vi "Global_Configurations.vi"() -> ()   [LabVIEW 2019]
panel:
  in  "LabVIEW Port":u16=3363 caption="SSE_frequency"
  in  "LabVIEW Host":string="localhost"
  in  "Session_timeout":u32=14400000
  in  "Reconnect_session_timeout":u32=12000
  in  "SSE_frequency":u32=200
  in  "Timeout_to abort_a_nonresponding_VI":u32=5000
  in  "License":cluster{"ID":string, "Number":string}
  in  "Access-Control-Allow-Credentials":string(combo)="true"
  out "VI_Disconnections":u8[](array[numeric])
  out "VI_Connections":u8[](array[numeric])
  in  "Access-Control-Allow-Origin":string
  in  "Default Experience":string="TestOK"
  in  "Base URL":string
  in  "Experiments":T1(array[cluster])=[{"Path"=path "../Private/TestOK.vi", "Name"="TestOK", "Authors"="D.Chaos", "Keywords"="Test", "Description"="TestOK.vi is used to test the correct execution of a well-defined vi through RIP", "Cameras"=[{"Base URL"="http://camera1_ip", "Path"="/axis-cgi/mjpg/video.cgi", "Name"="Camera 1"}, {"Base URL"="http://camera2_ip", "Path"="/axis-cgi/mjpg/video.cgi", "Name"="Camera 2"}], "Sampling"=[{"Sampled Variable"="t", "Delta"=5.0}], "Sampling Freq"=200}, {"Path"=path "C:/Users/Luis de la Torre/Documents/TestOK.vi", "Name"="TestOK2", "Authors"="D.Chaos", "Keywords"="Test", "Description"="TestOK.vi is used to test the correct execution of a well-defined vi through RIP", "Cameras"=[{"Base URL"="http://camera1_ip", "Path"="/axis-cgi/mjpg/video.cgi", "Name"="Camera 1"}, {"Base URL"="http://camera2_ip", "Path"="/axis-cgi/mjpg/video.cgi", "Name"="Camera 2"}], "Sampling"=[{"Sampled Variable"="t", "Delta"=5.0}], "Sampling Freq"=200}, {"Path"=path "C:/TestOK.vi", "Name"="TestOK3", "Authors"="D.Chaos", "Keywords"="Test", "Description"="TestOK.vi is used to test the correct execution of a well-defined vi through RIP", "Cameras"=[{"Base URL"="http://camera1_ip", "Path"="/axis-cgi/mjpg/video.cgi", "Name"="Camera 1"}, {"Base URL"="http://camera2_ip", "Path"="/axis-cgi/mjpg/video.cgi", "Name"="Camera 2"}], "Sampling"=[{"Sampled Variable"="t", "Delta"=5.0}], "Sampling Freq"=200}, {"Path"=path "../Private/TestDoNotClose.vi", "Name"="TestNO_STOP", "Authors"="D.Chaos", "Keywords"="Test", "Description"="TestDoNotClose.vi is used to test if RIP can automatically close a vi that never ends by itself", "Cameras"=[{"Base URL"="http://camera1_ip", "Path"="/axis-cgi/mjpg/video.cgi", "Name"="Camera 1"}], "Sampling"=[], "Sampling Freq"=200}]
  # "In order to save the configuration:\n1) Go to menu Edit/Make Current Values Default\n2) File/save"
  # "TODO: SSE_frecuency should be called sampling frequency and may be\ndifferent for each experience --> move to the Experiments cluster below"
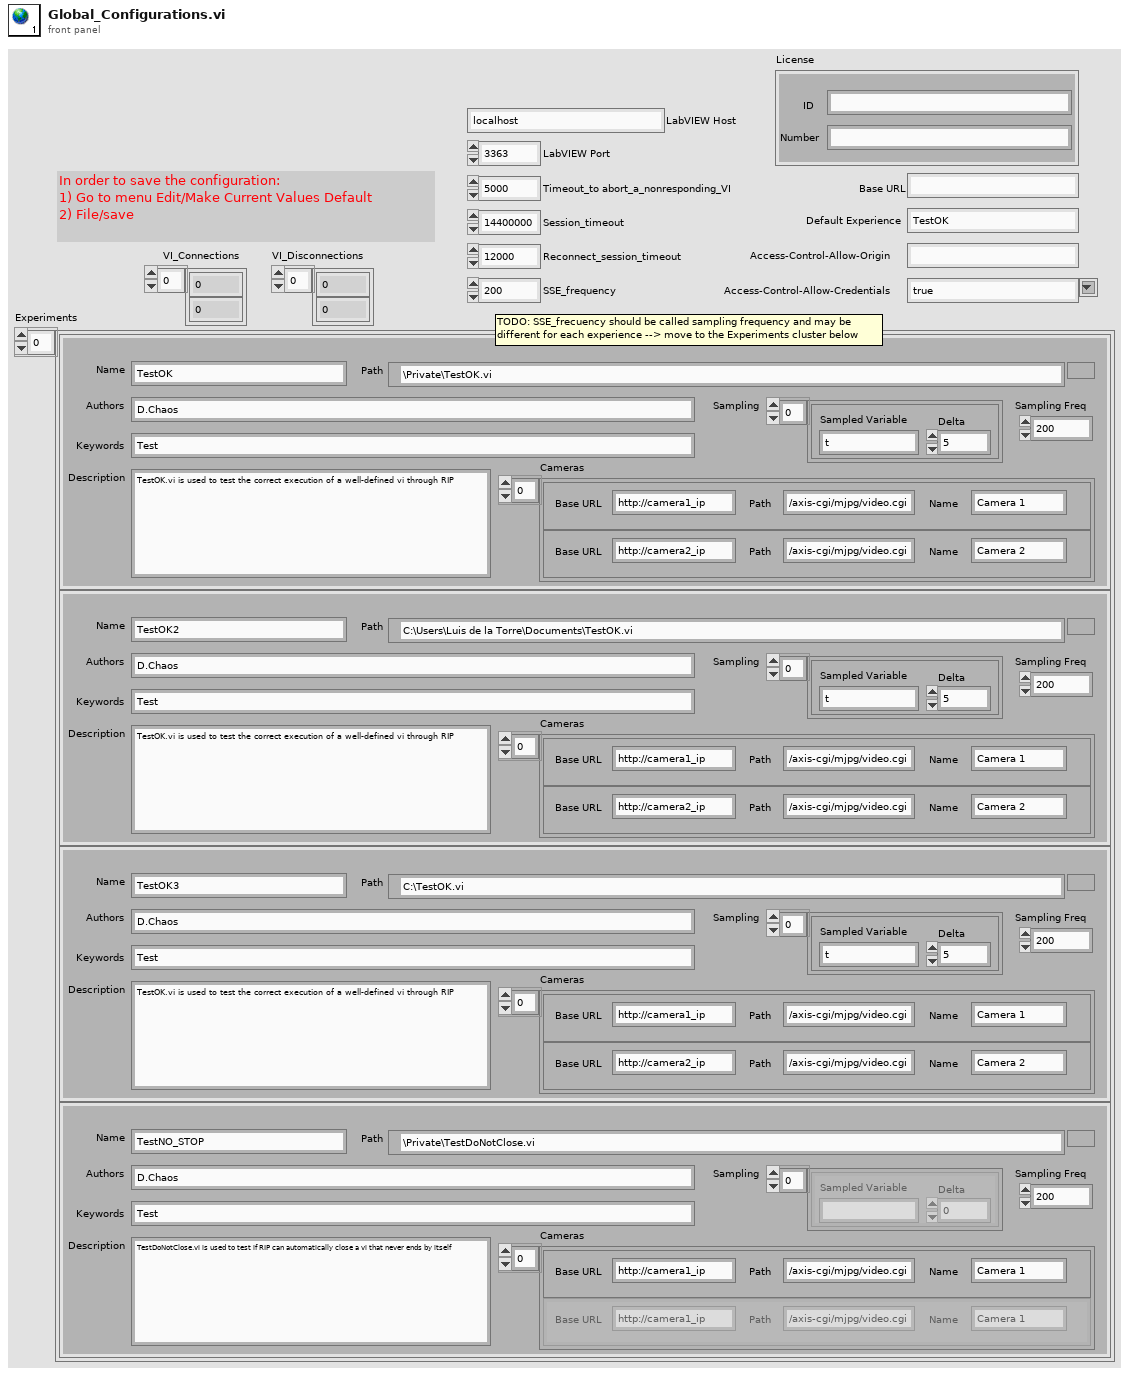
[diagram p1: front panel]
types:
  T1 = cluster{"Path":path, "Name":string, "Authors":string, "Keywords":string, "Description":string, "Cameras":cluster{"Base URL":string, "Path":string, "Name":string}[], "Sampling":cluster{"Sampled Variable":string, "Delta":dbl}[], "Sampling Freq":u32}[]
diagram:
